vi "ep_Points in Window.vi"(8 "minimum points for peak search":dbl format="%#_13g", 9 "df":dbl format="%#_13g", 10 "window configuration":T2(array[cluster]), 11 "all spectra points":cluster{"frequency":dbl[], "magnitude":dbl[]}) -> (3 "points in window":T1(array[cluster]))   [LabVIEW 2014, in "NI_EP_Motor Monitoring.lvlib"]
uses:
  <vilib>/addons/Electrical Power/Motor Monitoring/NI_EP_Motor Monitoring.lvlib
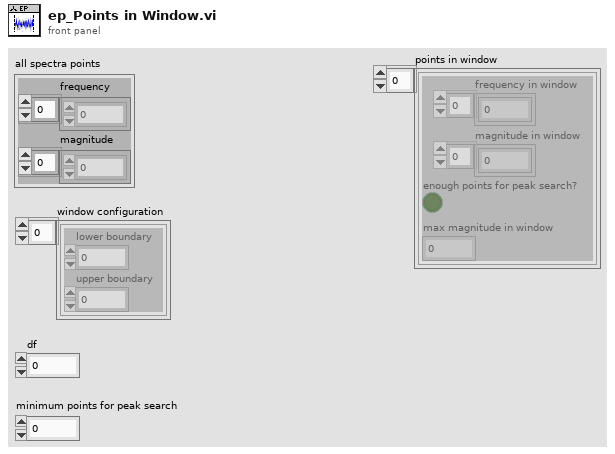
[diagram p1: front panel]
types:
  T1 = cluster{"frequency in window":dbl[], "magnitude in window":dbl[], "enough points for peak search?":bool, "max magnitude in window":dbl}[]
  T2 = cluster{"lower boundary":dbl, "upper boundary":dbl}[]
  T3 = cluster{"maximum frequency [Hz]":dbl, "slip error allowance":dbl, "minimum points for peak search":dbl, "accuracy of fs":dbl, "difference?":bool, " fs harmonics order":i32, "fs forbidden range":dbl, "p3:p1 valid significance ratio":dbl, "ratio for significance weighting":dbl, "significance weighting":dbl}
  T4 = cluster{"frequency in window":dbl[], "magnitude in window":dbl[], "enough points for peak search?":bool, "max magnitude in window":dbl}
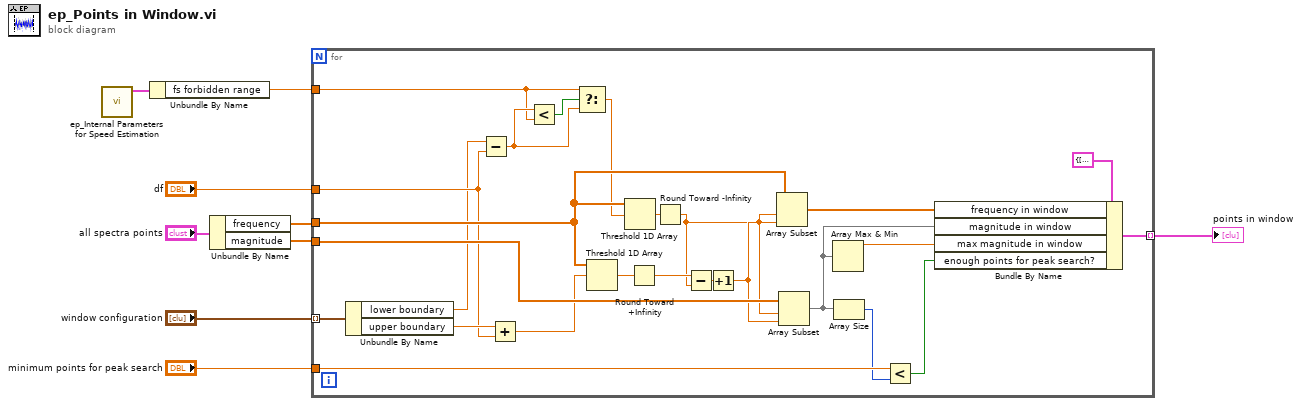
[diagram p0: block diagram]
diagram:
  n1 = call <vilib>:"ep_Internal Parameters for Speed Estimation.vi"() -> ("internal parameters for speed estimation"=w2:T3)  [unwired: 11 in]
  n2 = Unbundle By Name(w2) -> ("fs forbidden range"=w1:dbl)
  n3 = Unbundle By Name("all spectra points") -> ("frequency"=w5:dbl[], "magnitude"=w7:dbl[])
  n4 = for {
    tunnel: "window configuration" -> [w25] mode=indexing
    tunnel: w5 -> [w34]
    tunnel: w7 -> [w33]
    tunnel: "minimum points for peak search" -> [w27]
    tunnel: [w26] -> w4 mode=indexing
    tunnel: "df" -> [w21]
    tunnel: w1 -> [w15]
    n5 = Unbundle By Name(w25) -> ("lower boundary"=w19:dbl, "upper boundary"=w22:dbl)
    n6 = Subtract(x=w19, y=w21) -> (x-y=w17:dbl)
    n7 = Add(x=w22, y=w21) -> (x+y=w23:dbl)
    n8 = Less?(x=w17, y=w15) -> (x < y?=w20:bool)
    n9 = Select(t=w15, s=w20, f=w17) -> (s? t:f=w16:dbl)
    n10 = Threshold 1D Array(2:w23, 3:w34) -> (0:w31:dbl)  [unwired: 1 in]
    n11 = Threshold 1D Array(2:w16, 3:w34) -> (0:w32:dbl)  [unwired: 1 in]
    n12 = Round Toward +Infinity(x=w31) -> (ceil(x): smallest int >= x=w30:dbl)
    n13 = Round Toward -Infinity(1:w32) -> (0:w18:dbl)
    n14 = Subtract(x=w30, y=w18) -> (x-y=w29:dbl)
    n15 = Increment(x=w29) -> (x+1=w28:dbl)
    n16 = Array Subset(array=w34, index=w18, length=w28) -> (w24:dbl[])
    n17 = Array Subset(array=w33, index=w18, length=w28) -> (w11:dbl[])
    n18 = Array Max & Min(array=w11) -> (max value=w10:dbl)  [unwired: 3 out]
    n19 = Array Size(array=w11) -> (size(s)=w14:i32)
    n20 = Less?(x=w27, y=w14) -> (x < y?=w12:bool)
    n21 = Bundle By Name(cluster=T4 {"frequency in window"=[], "magnitude in window"=[], "enough points for peak search?"=FALSE, "max magnitude in window"=0.0} ("window spectra points"), "frequency in window"=w24, "magnitude in window"=w11, "max magnitude in window"=w10, "enough points for peak search?"=w12) -> (w26:T4)
  }
  "points in window" <- w4
